vi "Test Filter Dashed Method.vi"(8 "error in (no error)":errorcluster, 11 "Test Case In":refnum<class "Filter Test.lvclass">) -> (0 "error out":errorcluster, 3 "Test Case Out":refnum<class "Filter Test.lvclass">)   [LabVIEW 2020, in "Filter Test.lvclass"]
uses:
  Filter Test.lvclass
  Filter Test.lvclass/Filter Test.ctl
  source/API/LUnit Test Suite/LUnit Test Suite.lvclass
  source/API/Test Suite Factory/Test Suite Factory.lvclass
  source/Support/Filters/Dashed Filter/Dashed Filter.lvclass
  d5324887-24cf-49f2-99b3-caecd7888f3d.vi
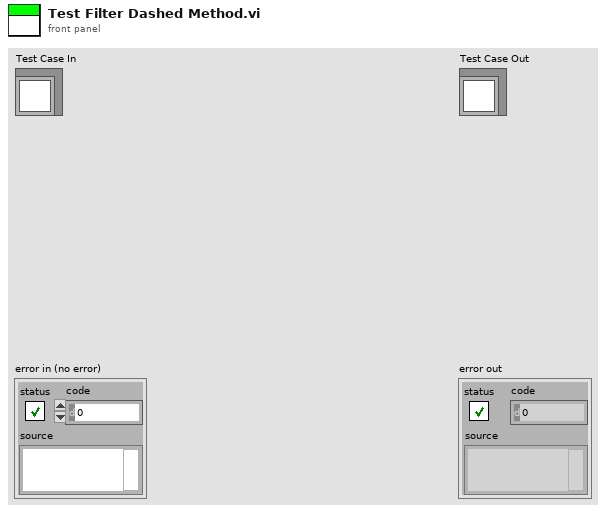
[diagram p1: front panel]
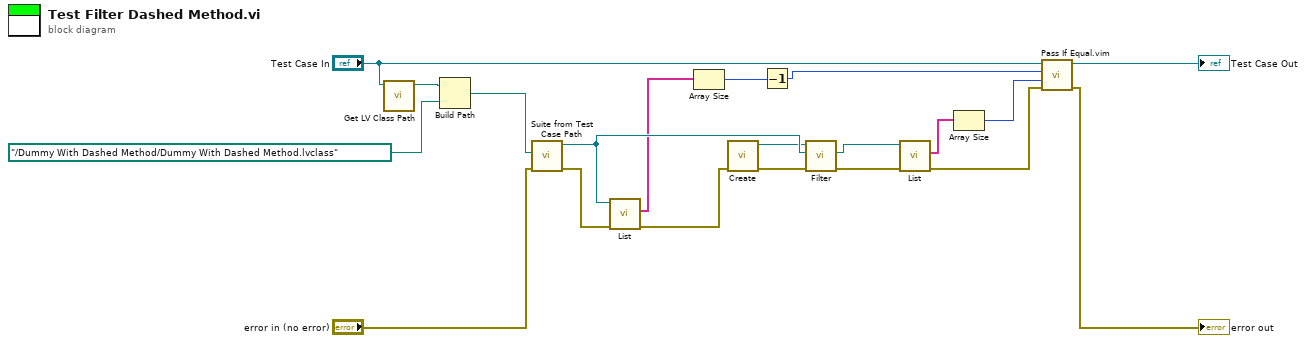
[diagram p0: block diagram]
diagram:
  n1 = call <vilib>:"Get LV Class Path.vi"("object"="Test Case In") -> ("class path"=w11:path)  [unwired: 9 in, 1 out]
  n2 = Build Path(base path=w11, name or relative path=path "../Dummy With Dashed Method/Dummy With Dashed Method.lvclass") -> (appended path=w9:path)
  n3 = call "Suite from Test Case Path.vi"("error in (no error)"="error in (no error)", "Test Case"=w9) -> ("error out"=w18:errorcluster, "LUnit Test Suite Out"=w13:refnum<class "LUnit Test Suite.lvclass">)  [unwired: 8 in]
  n4 = call "List.vi"("error in (no error)"=w18, "LUnit Test Suite In"=w13) -> ("error out"=w7:errorcluster, "List of Runnables"=w4:string[])  [unwired: 8 in]
  n5 = Array Size(array=w4) -> (size(s)=w3:i32)
  n6 = call "Create.vi"("error in (no error)"=w7) -> ("error out"=w6:errorcluster, "Dashed Filter"=w8:refnum<class "Dashed Filter.lvclass">)  [unwired: 9 in]
  n7 = Decrement(x=w3) -> (x-1=w1:i32)
  n8 = call-dynamic "Filter.vi"("error in (no error)"=w6, "Test Suite"=w13, "Dashed Filter in"=w8) -> ("error out"=w16:errorcluster, "Filtered Test Suite"=w17:refnum<class "LUnit Test Suite.lvclass">)  [unwired: 7 in]
  n9 = call "List.vi"("error in (no error)"=w16, "LUnit Test Suite In"=w17) -> ("error out"=w15:errorcluster, "List of Runnables"=w5:string[])  [unwired: 8 in]
  n10 = Array Size(array=w5) -> (size(s)=w2:i32)
  n11 = call "Pass If Equal.vim"("error in (no error)"=w15, "Actual"=w2, "Expected"=w1, "LUnit Test Case In"="Test Case In") -> ("error out"=→"error out":errorcluster, "LUnit Test Case Out"=→"Test Case Out":refnum<class "Filter Test.lvclass">)  [unwired: 6 in]
